vi "Write Distance.vi"(8 "error in (no error)":errorcluster, 10 "Distance":i32, 11 "Picture Ring in":refnum<class "Node.lvclass">) -> (0 "error out":errorcluster, 3 "Picture Ring out":refnum<class "Node.lvclass">)   [LabVIEW 2019, in "Node.lvclass"]
uses:
  Node.lvclass
  Node.lvclass/Node.ctl
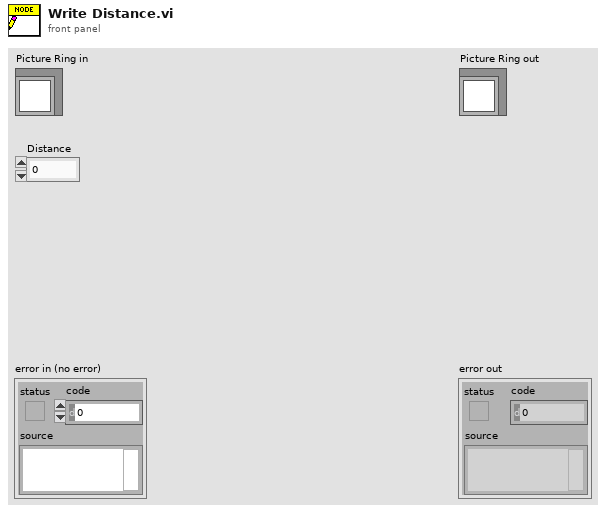
[diagram p1: front panel]
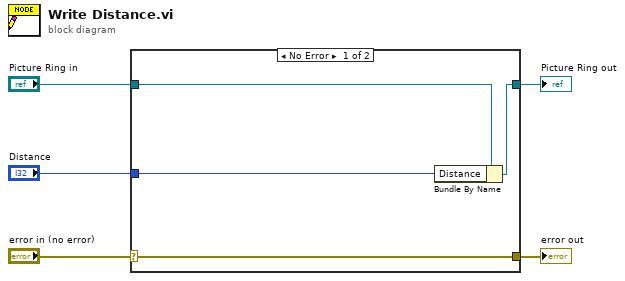
[diagram p0: block diagram]
diagram:
  n1 = case shown="No Error" "error in (no error)" {
    selector: "error in (no error)" -> [w9 w10]
    tunnel: [w9 w10] -> w4
    tunnel: [w7 w11] -> w2
    tunnel: "Picture Ring in" -> [w8 w11]
    tunnel: "Distance" -> [w6 _]
    frame No Error {
      n2 = Bundle By Name(cluster=w8, "Distance"=w6) -> (w7:refnum<class "Node.lvclass">)
    }
    frame Error {
    }
  }
  "error out" <- w4
  "Picture Ring out" <- w2
